vi "to string.vi"(8 "error in":errorcluster, 11 "Shared Library Module configuration in":refnum<class "Shared Library Module configuration.lvclass">) -> (0 "error out":errorcluster, 1 "data":string, 2 "version":string, 3 "Shared Library Module configuration out":refnum<class "Shared Library Module configuration.lvclass">)   [LabVIEW 2013, in "Shared Library Module configuration.lvclass"]
doc: "Provides an interface for saving a module configuration to a file or other serialized data source. It is recommended that all children of this class store data in two sets--data required for its own initialization, and any data required for parent initialization--and that each implementation uses the <b>Call Parent Method</b> primitive to serialize parent information.Platypus Framework 1.0.1.60\nNI Systems Engineering - National Instruments"
uses:
  Shared Library Module configuration.lvclass
  <vilib>/NI/Tag Bus Module Framework/module configuration/TBM module configuration.lvclass
  Shared Library Module configuration.lvclass/Shared Library Module configuration.ctl
  current version.vi
  <vilib>/NI/Configuration Framework/serializable configuration/NISE_CEF_serializable configuration.lvclass
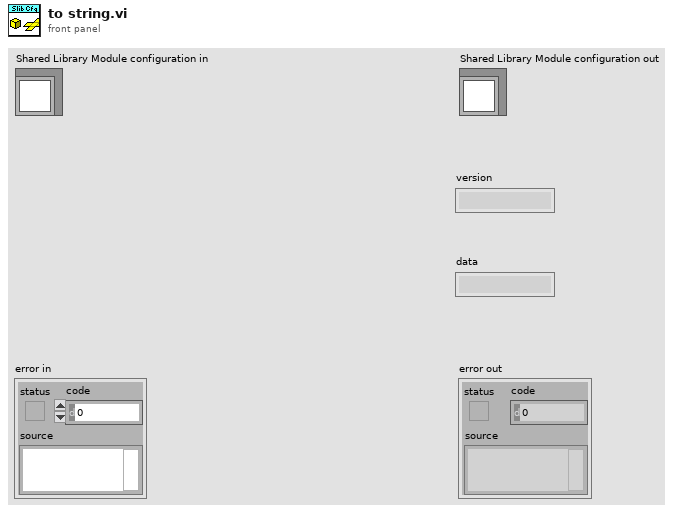
[diagram p1: front panel]
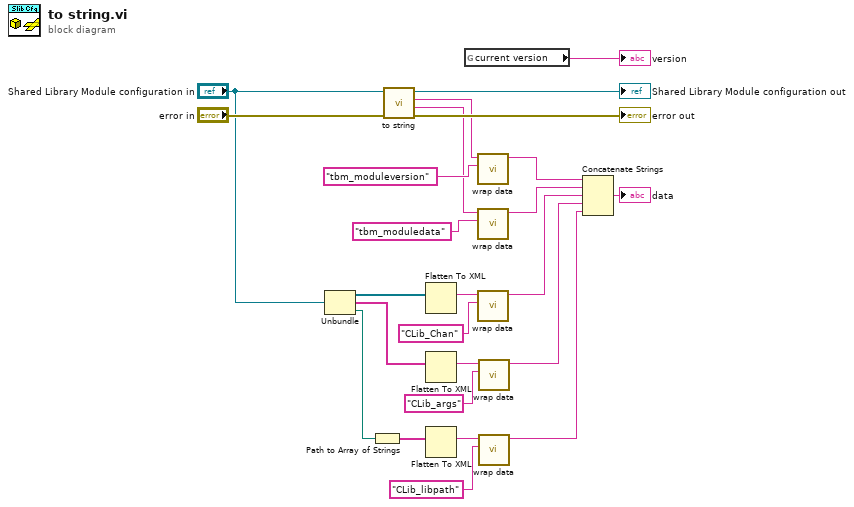
[diagram p0: block diagram]
diagram:
  n1 = Unbundle("Shared Library Module configuration in") -> (w17:refnum<class "TBM channel.lvclass">[], w10:string[], w9:path)
  n2 = Path to Array of Strings(0:w9) -> (2:w8:string[])  [unwired: 1 out]
  n3 = call-parent "to string.vi"("error in"="error in", "module configuration in"="Shared Library Module configuration in") -> ("error out"=→"error out":errorcluster, "data"=w1:string, "version"=w2:string, "module configuration out"=→"Shared Library Module configuration out":refnum<class "Shared Library Module configuration.lvclass">)  [unwired: 6 in]
  n4 = Flatten To XML(anything=w17) -> (xml string=w16:string)
  n5 = Flatten To XML(anything=w10) -> (xml string=w11:string)
  n6 = Flatten To XML(anything=w8) -> (xml string=w12:string)
  n7 = global read "current version.vi" "current version"() -> (→"version":string)
  n8 = call <vilib>:"wrap data.vi"("identifier"="tbm_moduleversion" ("additional identifier"), "data to wrap"=w2) -> ("wrapped data"=w19:string)  [unwired: 9 in]
  n9 = call <vilib>:"wrap data.vi"("identifier"="tbm_moduledata" ("additional identifier"), "data to wrap"=w1) -> ("wrapped data"=w18:string)  [unwired: 9 in]
  n10 = call <vilib>:"wrap data.vi"("identifier"="CLib_Chan" ("additional identifier"), "data to wrap"=w16) -> ("wrapped data"=w15:string)  [unwired: 9 in]
  n11 = call <vilib>:"wrap data.vi"("identifier"="CLib_args" ("additional identifier"), "data to wrap"=w11) -> ("wrapped data"=w13:string)  [unwired: 9 in]
  n12 = call <vilib>:"wrap data.vi"("identifier"="CLib_libpath" ("additional identifier"), "data to wrap"=w12) -> ("wrapped data"=w14:string)  [unwired: 9 in]
  n13 = Concatenate Strings(w19, w18, w15, w13, w14) -> (→"data":string)
